vi "Model - Set Config Data.vi"(8 "error in (no error)":errorcluster, 10 "Config Data":T1, 11 "View Model":T2) -> (0 "error out":errorcluster, 3 "View Model":T2)   [LabVIEW 2017]
doc: "Set current Config Data Array value to DVR."
uses:
  Controls/View Model.ctl
  Error Handler/Controls/Error Model.ctl
  Error Handler/Controls/Error Data.ctl
  Error Handler/Controls/Error Type.ctl
  Controls/Shared Model.ctl
  Configuration/Controls/Config Model.ctl
  Configuration/Controls/Config CMD.ctl
  Configuration/Controls/Config Data.ctl
  ATM Controller/Controls/Controller Model.ctl
  ATM Controller/Controls/Controller Overhead.ctl
  ATM Controller/Controls/Controller States.ctl
  ATM Controller/Controls/Controller Message Data.ctl
  ATM Controller/Controls/Controller Message Name.ctl
  ATM Controller/Controls/Controller CMD.ctl
  Views/User Console View/Controls/User Console - Transaction Enum.ctl
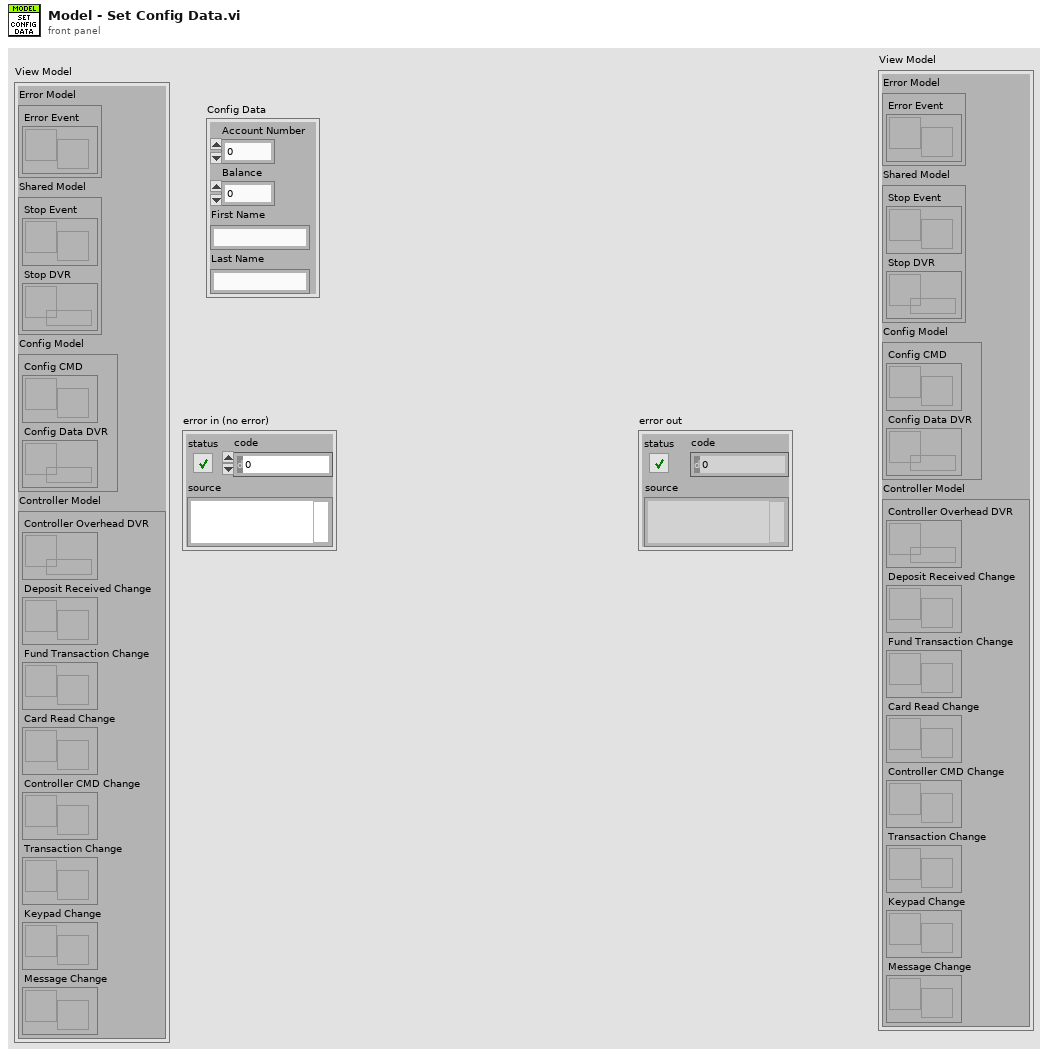
[diagram p1: front panel]
types:
  T1 = typedef "Config Data.ctl" = cluster{"Account Number":i32, "Balance":dbl, "First Name":string, "Last Name":string}
  T2 = typedef "View Model.ctl" = cluster{"Error Model":T3, "Shared Model":T4, "Config Model":T5, "Controller Model":T6}
  T3 = typedef "Error Model.ctl" = cluster{"Error Event":refnum<user-event>}
  T4 = typedef "Shared Model.ctl" = cluster{"Stop Event":refnum<user-event>, "Stop DVR":refnum<data-value>}
  T5 = typedef "Config Model.ctl" = cluster{"Config CMD":refnum<user-event>, "Config Data DVR":refnum<data-value>}
  T6 = typedef "Controller Model.ctl" = cluster{"Controller Overhead DVR":refnum<data-value>, "Deposit Received Change":refnum<user-event>, "Fund Transaction Change":refnum<user-event>, "Card Read Change":refnum<user-event>, "Controller CMD Change":refnum<user-event>, "Transaction Change":refnum<user-event>, "Keypad Change":refnum<user-event>, "Message Change":refnum<user-event>}
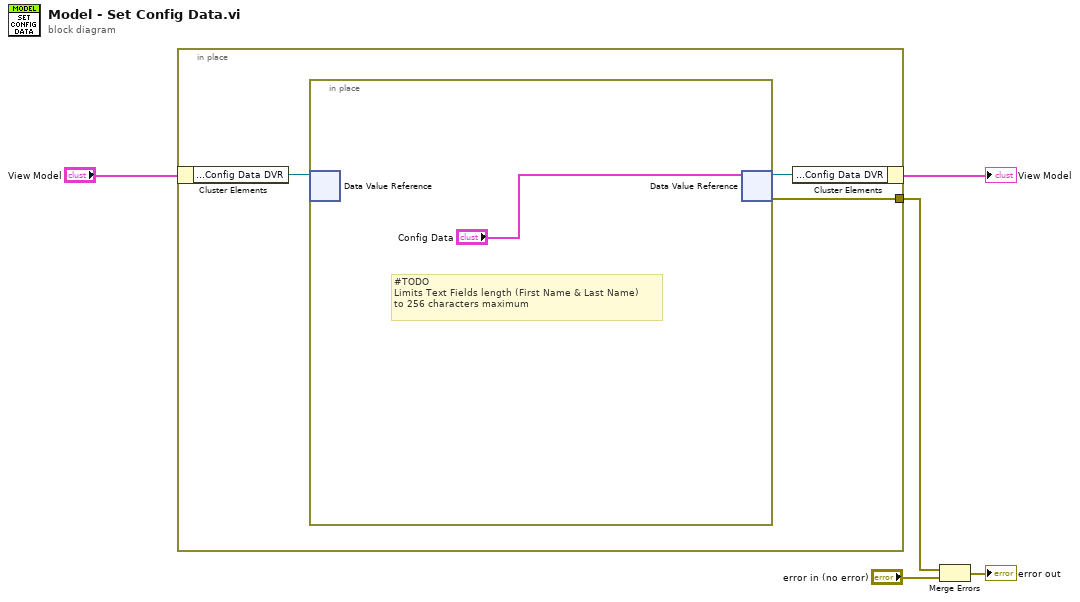
[diagram p0: block diagram]
diagram:
  n1 = in-place {
    in-place-border: [w6] -> w2
    n2 = in-place-cluster #1("View Model") -> ("Config Model.Config Data DVR"=w8:refnum<data-value>)
    n3 = in-place {
      # "#TODO\nLimits Text Fields length (First Name & Last Name)\nto 256 characters maximum"
      n4 = in-place-dvr #2(w8) -> ()  [unwired: 2 out]
      n5 = in-place-dvr #2("Config Data") -> (w7:refnum<data-value>, w6:errorcluster)
    }
    n6 = in-place-cluster #1("Config Model.Config Data DVR"=w7) -> (→"View Model":T2)
  }
  n7 = Merge Errors(w2, "error in (no error)") -> (→"error out":errorcluster)
